vi "Auto Intake.vi"(0 "Intake Mode ID":i32, 1 "Intake Command ID":i32, 2 "Arm Angle":dbl, 5 "Intake Override Speed":dbl, 7 "Eject Override Speed":dbl, 9 "Arm Speed":dbl, 10 "Override Intake?":i32, 11 "Intake?":i32, 12 "Override Eject?":i32, 13 "Override Angle?":i32, 14 "Override Arm?":i32, 15 "Eject?":i32) -> ()   [LabVIEW 2015]
uses:
  Common Code/Intake Mode.ctl
  Common Code/Intake Commands.ctl
  Robot Global Data.vi
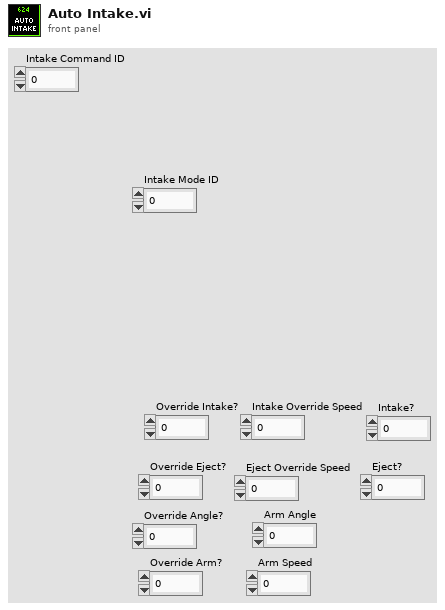
[diagram p1: front panel]
types:
  T1 = typedef "Intake Mode.ctl" = enum16{"Manual", "Safe", "Auto"}
  T2 = typedef "Intake Commands.ctl" = enum16{"Zero", "Unload", "Load", "Drop low", "Idle"}
  T3 = typedef "Manual Intake Commands.ctl" = cluster{"Intake":bool, "Eject":bool, "Arm Angle":dbl, "Intake Override Speed":dbl, "Arm Override Speed":dbl, "Arm Speed":dbl, "Override Intake":bool, "Override Eject":bool, "Eject Override Speed":dbl, "Arm":bool, "Override Arm":bool, "Override Angle":bool}
  T4 = typedef "Intake Commands Cluster.ctl" = cluster{"Intake Commands":T2, "Intake Mode":T1}
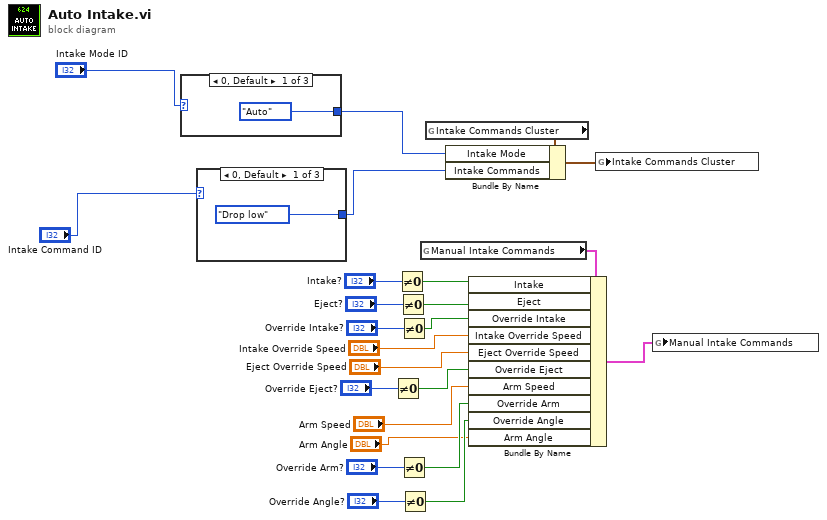
[diagram p0: block diagram]
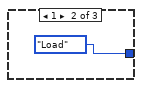
[diagram p2: hidden frame]
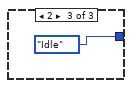
[diagram p3: hidden frame]
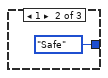
[diagram p4: hidden frame]
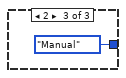
[diagram p5: hidden frame]
diagram:
  n1 = case shown="0, Default" "Intake Mode ID" {
    tunnel: [Intake_Mode."Auto" ("Intake Mode") Intake_Mode."Safe" ("Intake Mode") Intake_Mode."Manual" ("Intake Mode")] -> w21
    frame 0, Default {
    }
    frame 1 {
    }
    frame 2 {
    }
  }
  n2 = case shown="0, Default" "Intake Command ID" {
    tunnel: [Intake_Commands."Drop low" ("Intake Commands") Intake_Commands."Load" ("Intake Commands") Intake_Commands."Idle" ("Intake Commands")] -> w2
    frame 0, Default {
    }
    frame 1 {
    }
    frame 2 {
    }
  }
  n3 = Not Equal To 0?(x="Override Eject?") -> (x != 0?=w9:bool)
  n4 = Not Equal To 0?(x="Intake?") -> (x != 0?=w17:bool)
  n5 = Not Equal To 0?(x="Eject?") -> (x != 0?=w15:bool)
  n6 = Not Equal To 0?(x="Override Intake?") -> (x != 0?=w13:bool)
  n7 = Not Equal To 0?(x="Override Arm?") -> (x != 0?=w6:bool)
  n8 = Not Equal To 0?(x="Override Angle?") -> (x != 0?=w4:bool)
  n9 = global read "Robot Global Data.vi" "Manual Intake Commands"() -> (w20:T3)
  n10 = global read "Robot Global Data.vi" "Intake Commands Cluster"() -> (w23:T4)
  n11 = Bundle By Name(cluster=w23, "Intake Mode"=w21, "Intake Commands"=w2) -> (w24:T4)
  n12 = Bundle By Name(cluster=w20, "Intake"=w17, "Eject"=w15, "Override Intake"=w13, "Intake Override Speed"="Intake Override Speed", "Eject Override Speed"="Eject Override Speed", "Override Eject"=w9, "Arm Speed"="Arm Speed", "Override Arm"=w6, "Override Angle"=w4, "Arm Angle"="Arm Angle") -> (w19:T3)
  n13 = global write "Robot Global Data.vi" "Intake Commands Cluster"(w24) -> ()
  n14 = global write "Robot Global Data.vi" "Manual Intake Commands"(w19) -> ()
